vi "roboRIO v1.0 Unreserve Channel.vi"(5 "Allow multiple opens?":bool, 7 "Owner":string, 8 "error in (no error)":errorcluster, 9 "Mutex ID":i32, 10 "Connector":T1=enum."ConnectorB", 11 "Channel Name":string) -> (0 "error out":errorcluster)   [LabVIEW 2021]
uses:
  <vilib>/myRIO/Common/Instrument Driver Framework/roboRIO v1.0/Resource Manager/typedefs/roboRIO v1.0 Connector List.ctl
  <vilib>/myRIO/Common/Instrument Driver Framework/Utilities/typedefs/Resource Manager Action Enum.ctl
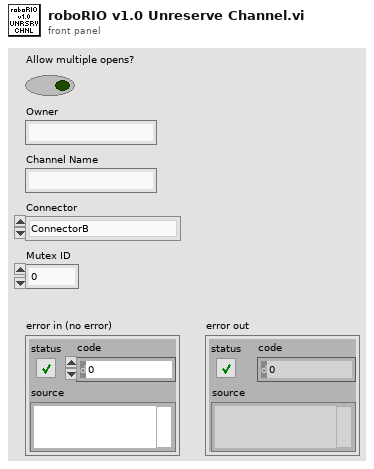
[diagram p1: front panel]
types:
  T1 = typedef "roboRIO v1.0 Connector List.ctl" = enum32{"None", "ConnectorB", "ConnectorI2C", "ConnectorDIO", "ConnectorRSL", "ConnectorRELAY", "ConnectorAI", "ConnectorPWM", "ConnectorSPI"}
  T2 = typedef "Resource Manager Action Enum.ctl" = enum16{"Lock", "Unlock"}
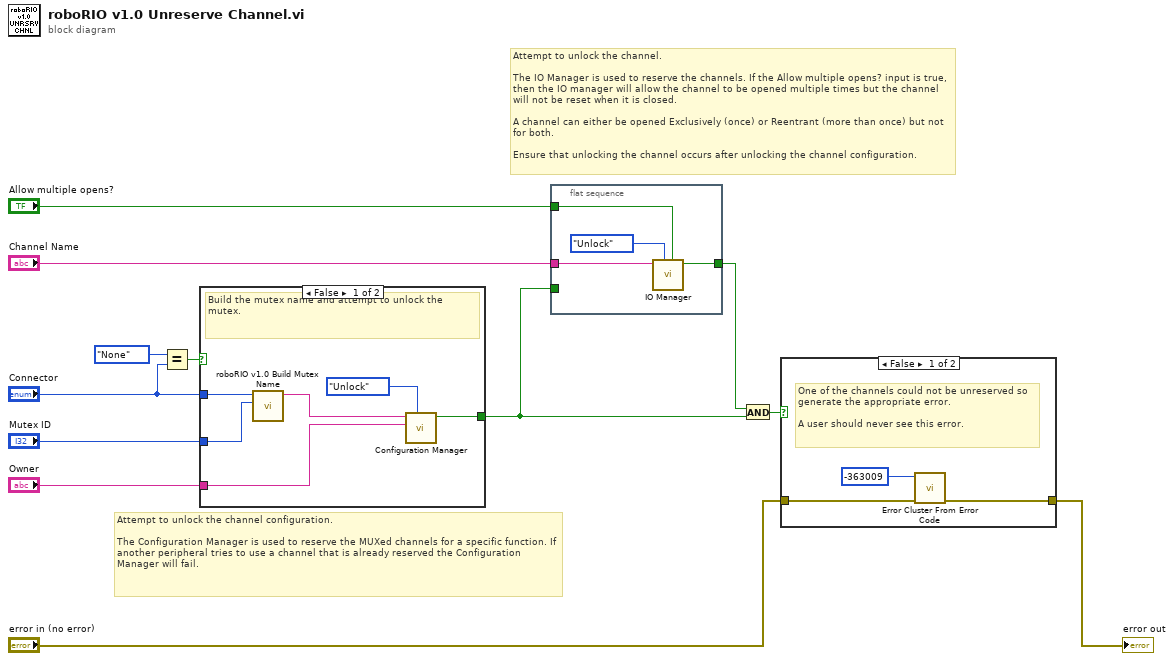
[diagram p0: block diagram]
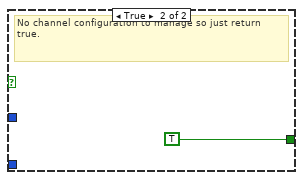
[diagram p3: hidden frame]
diagram:
  # "Attempt to unlock the channel configuration.\n\nThe Configuration Manager is used to reserve the MUXed channels for a specific function. If another peripheral tries to use a channel that is already reserved the Configuration Manager will fail."
  # "Attempt to unlock the channel.\n\nThe IO Manager is used to reserve the channels. If the Allow multiple opens? input is true, then the IO manager will allow the channel to be opened multiple times but the channel will not be reset when it is closed.\n\nA channel can either be opened Exclusively (once) or Reentrant (more than once) but not for both.\n\nEnsure that unlocking the channel occurs after unlocking the channel configuration."
  n1 = Equal?(x=roboRIO_v1.0_Connector_List."None" ("y"), y="Connector") -> (x = y?=w6:bool)
  n2 = case shown="False" w6 {
    tunnel: [w16 TRUE ("Reentrant?")] -> w4
    tunnel: "Owner" -> [w18 _]
    tunnel: "Connector" -> [w15 _]
    tunnel: "Mutex ID" -> [w14 _]
    frame False {
      # "Build the mutex name and attempt to unlock the mutex."
      n3 = call <vilib>:"roboRIO v1.0 Build Mutex Name.vi"("Mutex ID"=w14, "Connector"=w15) -> ("Mutex Name"=w13:string)  [unwired: 9 in]
      n4 = call <vilib>:"Configuration Manager.vi"("Actions"=Resource_Manager_Action_Enum."Unlock", "Owner"=w18, "Mutex Name"=w13) -> ("Success?"=w16:bool)  [unwired: 8 in]
    }
    frame True {
      # "No channel configuration to manage so just return true."
    }
  }
  n5 = flat-sequence {
    tunnel: "Allow multiple opens?" -> [w23]
    tunnel: "Channel Name" -> [w22]
    tunnel: [w21] -> w5
    tunnel: w4 -> [_]
    frame #0 {
      n6 = call <vilib>:"IO Manager.vi"("Reentrant?"=w23, "Actions"=Resource_Manager_Action_Enum."Unlock", "Mutex Name"=w22) -> ("Success?"=w21:bool)  [unwired: 8 in]
    }
  }
  n7 = And(x=w5, y=w4) -> (x .and. y?=w3:bool)
  n8 = case shown="False" w3 {
    tunnel: "error in (no error)" -> [w26 w27]
    tunnel: [w25 w27] -> w1
    frame False {
      # "One of the channels could not be unreserved so generate the appropriate error.\n\nA user should never see this error."
      n9 = call <vilib>:"Error Cluster From Error Code.vi"("error in (no error)"=w26, "error code (0)"=-363009) -> ("error out"=w25:errorcluster)  [unwired: 7 in]
    }
    frame True {
    }
  }
  "error out" <- w1
